vi "Connect.vi"(8 "error in (no error)":errorcluster, 10 "Addon Name":string, 11 "Address":string) -> (0 "error out":errorcluster, 3 "Ref":T1)   [LabVIEW 2019, in "Protection and Counter Host Automation API.lvlib"]
uses:
  Protection and Counter Host Automation API.lvlib
  Types/API Variables.ctl
  <vilib>/NI/STM/TCP/TCP Connection Info.ctl
  <vilib>/NI/STM/SubVIs/MetaDataElement.ctl
  <vilib>/NI/STM/TCP/Write Meta Data (TCP Ref).vi
  <vilib>/NI/STM/TCP/Write Meta Data (TCP Clst).vi
  <vilib>/NI/STM/NI STM.lvlib
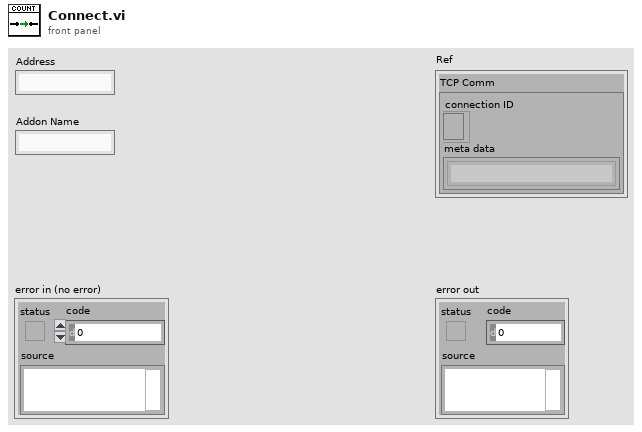
[diagram p1: front panel]
types:
  T1 = typedef "Protection and Counter Host Automation API.lvlib/API Variables.ctl" = cluster{"TCP Comm":T2}
  T2 = typedef "NI STM.lvlib/TCP Connection Info.ctl" = cluster{"connection ID":refnum<k5>, "meta data":T3[]}
  T3 = typedef "NI STM.lvlib/MetaDataElement.ctl" = string
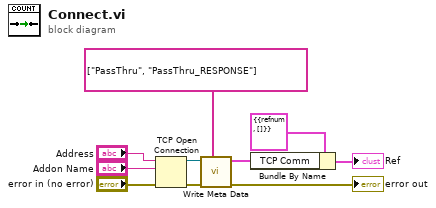
[diagram p0: block diagram]
diagram:
  n1 = TCP Open Connection(address="Address", remote port or service name="Addon Name", error in (no error)="error in (no error)") -> (connection ID=w9:refnum<k5>, error out=w10:errorcluster)  [unwired: 2 in]
  n2 = call-poly <vilib>:"Write Meta Data.vi"("meta data"=string[] ["PassThru", "PassThru_RESPONSE"] ("Meta data"), "error in"=w10, "connection ID"=w9) -> ("error out"=→"error out":errorcluster, "connection info out"=w2:T2)  [unwired: 7 in]
  n3 = Bundle By Name(cluster=T1 {"TCP Comm"={"connection ID"=refnum, "meta data"=[]}} ("Ref 2"), "TCP Comm"=w2) -> (→"Ref":T1)
